vi "1_PatchCore_Eval.vi"(0 "Trained_Model_Paths":T6={"NNFE_Paths"={"CFG"=path "D:/bottle__25_02_07__21_20_24/bottle_NNFE__25_02_07__21_20_24.cfg", "BIN"=path "D:/bottle__25_02_07__21_20_24/bottle_NNFE__25_02_07__21_20_24.bin"}, "PatchCore_Paths"={"CFG"=path "D:/bottle__25_02_07__21_20_24/bottle_Patchcore__25_02_07__21_20_24.cfg", "BIN"=path "D:/bottle__25_02_07__21_20_24/bottle_MemBank__PS3_RP296_SR0.1_Size16.4k__25_02_07__21_20_24.bin"}}, 1 "NNFE_CFG":T10={"Input_Dims"={"C"=-1, "H"=-1, "W"=-1}, "mBatch"=1}, 3 "Feature_Scorer_Params":T8={"Nearest_Neihbours"=1, "Calculate Anomaly Map"=TRUE, "Gaussian_Blur"={"Kernel_Size"=33, "sigma"=4.0}}, 7 "Dataset_Path(Validation)":path=path "D:/MVTec/bottle/test", 9 "Ground_Truth_Folder_Path":path=path "D:/MVTec/bottle/ground_truth", 11 "error in":errorcluster, 12 "Device_Config.":T4={"Device"=enum."GPU", "GPU Id"=0}) -> (4 "Eval_Stats_File_Path":path=path "D:/bottle__25_02_07__21_20_24/PatchCore_Eval_Stats__25_02_07__21_20_46.cfg", 13 "Evaluation_Metrics(Pixel)":T1={"Scores(Good)"={"X Values"=[2.5187396848201753, 3.240138484239578, 3.9615372836589815, 4.682936083078385, 5.404334882497787, 6.125733681917191, 6.847132481336594, 7.568531280755996, 8.289930080175399, 9.011328879594803, 9.732727679014207, 10.454126478433608, 11.175525277853012, 11.896924077272416, 12.618322876691819, 13.339721676111221, 14.061120475530625, 14.782519274950028, 15.50391807436943, 16.225316873788834, 16.94671567320824, 17.668114472627643, 18.389513272047044, 19.110912071466444, 19.83231087088585, 20.553709670305253, 21.275108469724657, 21.99650726914406, 22.71790606856346, 23.439304867982866, 24.160703667402267, 24.88210246682167, 25.603501266241075, 26.32490006566048, 27.04629886507988, 27.767697664499284, 28.489096463918685, 29.21049526333809, 29.931894062757493, 30.653292862176897, 31.3746916615963, 32.096090461015706, 32.81748926043511, 33.538888059854514, 34.26028685927391, 34.981685658693316, 35.70308445811272, 36.42448325753212, 37.14588205695152, 37.867280856370925, 38.58867965579033, 39.310078455209734, 40.03147725462914, 40.75287605404854, 41.474274853467946, 42.19567365288734, 42.91707245230675, 43.63847125172615, 44.359870051145556, 45.08126885056496, 45.80266764998436, 46.52406644940376, 47.245465248823166, 47.96686404824257, 48.688262847661974, 49.40966164708138, 50.13106044650078, 50.85245924592019, 51.573858045339584, 52.29525684475899, 53.01665564417839, 53.7380544435978, 54.4594532430172, 55.1808520424366, 55.902250841856, 56.62364964127541, 57.34504844069481, 58.066447240114215, 58.78784603953362, 59.50924483895302, 60.23064363837243, 60.952042437791825, 61.67344123721123, 62.39484003663063, 63.11623883605004, 63.83763763546945, 64.55903643488884, 65.28043523430824, 66.00183403372765, 66.72323283314705, 67.44463163256646, 68.16603043198586, 68.88742923140526, 69.60882803082467, 70.33022683024407, 71.05162562966348, 71.77302442908287, 72.49442322850227, 73.21582202792167, 73.93722082734108], "Histogram: h(x)"=[90, 939, 2938, 5870, 8902, 11734, 15274, 18341, 21048, 26598, 31500, 33798, 32899, 32682, 35302, 38511, 44001, 47200, 57146, 83639, 108421, 109082, 88841, 61245, 37236, 23127, 12524, 6486, 3678, 1409, 910, 781, 568, 237, 213, 141, 123, 86, 0, 0, 0, 0, 0, 0, 0, 0, 0, 0, 0, 0, 0, 0, 0, 0, 0, 0, 0, 0, 0, 0, 0, 0, 0, 0, 0, 0, 0, 0, 0, 0, 0, 0, 0, 0, 0, 0, 0, 0, 0, 0, 0, 0, 0, 0, 0, 0, 0, 0, 0, 0, 0, 0, 0, 0, 0, 0, 0, 0, 0, 0]}, "Scores(Bad)"={"X Values"=[2.5187396848201753, 3.240138484239578, 3.9615372836589815, 4.682936083078385, 5.404334882497787, 6.125733681917191, 6.847132481336594, 7.568531280755996, 8.289930080175399, 9.011328879594803, 9.732727679014207, 10.454126478433608, 11.175525277853012, 11.896924077272416, 12.618322876691819, 13.339721676111221, 14.061120475530625, 14.782519274950028, 15.50391807436943, 16.225316873788834, 16.94671567320824, 17.668114472627643, 18.389513272047044, 19.110912071466444, 19.83231087088585, 20.553709670305253, 21.275108469724657, 21.99650726914406, 22.71790606856346, 23.439304867982866, 24.160703667402267, 24.88210246682167, 25.603501266241075, 26.32490006566048, 27.04629886507988, 27.767697664499284, 28.489096463918685, 29.21049526333809, 29.931894062757493, 30.653292862176897, 31.3746916615963, 32.096090461015706, 32.81748926043511, 33.538888059854514, 34.26028685927391, 34.981685658693316, 35.70308445811272, 36.42448325753212, 37.14588205695152, 37.867280856370925, 38.58867965579033, 39.310078455209734, 40.03147725462914, 40.75287605404854, 41.474274853467946, 42.19567365288734, 42.91707245230675, 43.63847125172615, 44.359870051145556, 45.08126885056496, 45.80266764998436, 46.52406644940376, 47.245465248823166, 47.96686404824257, 48.688262847661974, 49.40966164708138, 50.13106044650078, 50.85245924592019, 51.573858045339584, 52.29525684475899, 53.01665564417839, 53.7380544435978, 54.4594532430172, 55.1808520424366, 55.902250841856, 56.62364964127541, 57.34504844069481, 58.066447240114215, 58.78784603953362, 59.50924483895302, 60.23064363837243, 60.952042437791825, 61.67344123721123, 62.39484003663063, 63.11623883605004, 63.83763763546945, 64.55903643488884, 65.28043523430824, 66.00183403372765, 66.72323283314705, 67.44463163256646, 68.16603043198586, 68.88742923140526, 69.60882803082467, 70.33022683024407, 71.05162562966348, 71.77302442908287, 72.49442322850227, 73.21582202792167, 73.93722082734108], "Histogram: h(x)"=[0, 0, 0, 0, 0, 0, 0, 0, 0, 0, 0, 0, 0, 0, 0, 0, 0, 0, 0, 0, 0, 0, 0, 0, 3, 18, 4, 4, 22, 166, 350, 529, 712, 1080, 1390, 2090, 2510, 2735, 2990, 3683, 3643, 4025, 4368, 4354, 5075, 4848, 4451, 4310, 4479, 4659, 4932, 5114, 5826, 5988, 5477, 5336, 5670, 5902, 6292, 7002, 6961, 7000, 6738, 6629, 6889, 6684, 6682, 6438, 6484, 6148, 6044, 5899, 5338, 5008, 4726, 4469, 4002, 3233, 2677, 2298, 2183, 1919, 1568, 1056, 735, 519, 423, 414, 455, 561, 433, 377, 366, 353, 270, 185, 83, 74, 69, 64]}, "Eval Stats"={"Scores(Good)"={"Min"=2.1580403, "Max"=29.366932}, "Scores(Bad)"={"Min"=19.911945, "Max"=74.29792}, "# of Samples(Good)"=1003520, "# of Samples(Bad)"=242491, "AUROC"=0.9999726, "F1_Max"=0.994964, "Thrshld(F1_Max)"=25.554758, "Prec.(F1_Max)"=0.99552876, "Recall(F1_Max)"=0.9943998, "FPR(F1_Max)"=0.0010792012, "FNR(F1_Max)"=0.005600208}} {"Eval Stats"."Recall(F1_Max)" format="%#.5f"; "Eval Stats"."FPR(F1_Max)" format="%#.5f"; "Eval Stats"."FNR(F1_Max)" format="%#.5f"; "Eval Stats"."Prec.(F1_Max)" format="%#.5f"; "Eval Stats"."F1_Max" format="%#.5f"; "Eval Stats"."AUROC" format="%#.5f"; "Eval Stats"."Scores(Bad)"."Min" format="%#_5g"; "Eval Stats"."Scores(Good)"."Min" format="%#_5g"; "Eval Stats"."Thrshld(F1_Max)" format="%#_5f"}, 14 "Evaluation_Metrics(Image)":T1={"Scores(Good)"={"X Values"=[21.021667575836183, 21.57413511276245, 22.12660264968872, 22.679070186614993, 23.23153772354126, 23.78400526046753, 24.336472797393796, 24.88894033432007, 25.44140787124634, 25.993875408172606, 26.54634294509888, 27.098810482025144, 27.651278018951416, 28.203745555877685, 28.756213092803954, 29.308680629730226, 29.86114816665649, 30.413615703582764, 30.966083240509032, 31.5185507774353, 32.071018314361574, 32.62348585128784, 33.17595338821411, 33.728420925140384, 34.28088846206665, 34.83335599899292, 35.38582353591919, 35.93829107284546, 36.490758609771724, 37.043226146698, 37.59569368362427, 38.148161220550534, 38.70062875747681, 39.25309629440307, 39.805563831329344, 40.35803136825562, 40.91049890518188, 41.462966442108154, 42.01543397903442, 42.56790151596069, 43.120369052886964, 43.67283658981323, 44.2253041267395, 44.77777166366577, 45.33023920059204, 45.88270673751831, 46.43517427444458, 46.98764181137085, 47.540109348297115, 48.09257688522339, 48.64504442214966, 49.197511959075925, 49.7499794960022, 50.30244703292846, 50.854914569854735, 51.407382106781, 51.95984964370727, 52.512317180633545, 53.06478471755981, 53.61725225448608, 54.16971979141235, 54.72218732833862, 55.27465486526489, 55.82712240219116, 56.37958993911743, 56.932057476043695, 57.48452501296997, 58.03699254989624, 58.589460086822506, 59.14192762374878, 59.69439516067504, 60.246862697601316, 60.79933023452759, 61.35179777145385, 61.904265308380126, 62.45673284530639, 63.00920038223266, 63.561667919158936, 64.1141354560852, 64.66660299301148, 65.21907052993774, 65.77153806686401, 66.32400560379028, 66.87647314071654, 67.42894067764283, 67.98140821456909, 68.53387575149536, 69.08634328842163, 69.63881082534789, 70.19127836227418, 70.74374589920043, 71.2962134361267, 71.84868097305298, 72.40114850997924, 72.95361604690552, 73.50608358383178, 74.05855112075805, 74.61101865768433, 75.16348619461058, 75.71595373153687], "Histogram: h(x)"=[1, 0, 0, 8, 2, 2, 0, 1, 1, 0, 0, 2, 1, 0, 0, 1, 0, 0, 1, 0, 0, 0, 0, 0, 0, 0, 0, 0, 0, 0, 0, 0, 0, 0, 0, 0, 0, 0, 0, 0, 0, 0, 0, 0, 0, 0, 0, 0, 0, 0, 0, 0, 0, 0, 0, 0, 0, 0, 0, 0, 0, 0, 0, 0, 0, 0, 0, 0, 0, 0, 0, 0, 0, 0, 0, 0, 0, 0, 0, 0, 0, 0, 0, 0, 0, 0, 0, 0, 0, 0, 0, 0, 0, 0, 0, 0, 0, 0, 0, 0]}, "Scores(Bad)"={"X Values"=[21.021667575836183, 21.57413511276245, 22.12660264968872, 22.679070186614993, 23.23153772354126, 23.78400526046753, 24.336472797393796, 24.88894033432007, 25.44140787124634, 25.993875408172606, 26.54634294509888, 27.098810482025144, 27.651278018951416, 28.203745555877685, 28.756213092803954, 29.308680629730226, 29.86114816665649, 30.413615703582764, 30.966083240509032, 31.5185507774353, 32.071018314361574, 32.62348585128784, 33.17595338821411, 33.728420925140384, 34.28088846206665, 34.83335599899292, 35.38582353591919, 35.93829107284546, 36.490758609771724, 37.043226146698, 37.59569368362427, 38.148161220550534, 38.70062875747681, 39.25309629440307, 39.805563831329344, 40.35803136825562, 40.91049890518188, 41.462966442108154, 42.01543397903442, 42.56790151596069, 43.120369052886964, 43.67283658981323, 44.2253041267395, 44.77777166366577, 45.33023920059204, 45.88270673751831, 46.43517427444458, 46.98764181137085, 47.540109348297115, 48.09257688522339, 48.64504442214966, 49.197511959075925, 49.7499794960022, 50.30244703292846, 50.854914569854735, 51.407382106781, 51.95984964370727, 52.512317180633545, 53.06478471755981, 53.61725225448608, 54.16971979141235, 54.72218732833862, 55.27465486526489, 55.82712240219116, 56.37958993911743, 56.932057476043695, 57.48452501296997, 58.03699254989624, 58.589460086822506, 59.14192762374878, 59.69439516067504, 60.246862697601316, 60.79933023452759, 61.35179777145385, 61.904265308380126, 62.45673284530639, 63.00920038223266, 63.561667919158936, 64.1141354560852, 64.66660299301148, 65.21907052993774, 65.77153806686401, 66.32400560379028, 66.87647314071654, 67.42894067764283, 67.98140821456909, 68.53387575149536, 69.08634328842163, 69.63881082534789, 70.19127836227418, 70.74374589920043, 71.2962134361267, 71.84868097305298, 72.40114850997924, 72.95361604690552, 73.50608358383178, 74.05855112075805, 74.61101865768433, 75.16348619461058, 75.71595373153687], "Histogram: h(x)"=[0, 0, 0, 0, 0, 0, 0, 0, 0, 0, 0, 0, 0, 0, 0, 0, 0, 0, 0, 0, 0, 0, 0, 0, 0, 1, 0, 0, 0, 1, 1, 1, 1, 0, 0, 1, 0, 0, 0, 0, 1, 1, 0, 0, 1, 0, 0, 0, 1, 2, 1, 0, 1, 0, 2, 2, 0, 0, 0, 0, 1, 0, 2, 3, 0, 4, 0, 0, 1, 2, 2, 2, 3, 2, 3, 4, 1, 2, 2, 2, 2, 0, 0, 1, 0, 2, 0, 0, 0, 0, 0, 0, 1, 0, 1, 0, 1, 0, 0, 1]}, "Eval Stats"={"Scores(Good)"={"Min"=20.745434, "Max"=30.757803}, "Scores(Bad)"={"Min"=34.900276, "Max"=75.99219}, "# of Samples(Good)"=20, "# of Samples(Bad)"=63, "AUROC"=1.0, "F1_Max"=1.0, "Thrshld(F1_Max)"=30.810408, "Prec.(F1_Max)"=1.0, "Recall(F1_Max)"=1.0, "FPR(F1_Max)"=0.0, "FNR(F1_Max)"=0.0}} {"Eval Stats"."Recall(F1_Max)" format="%#.5f"; "Eval Stats"."FPR(F1_Max)" format="%#.5f"; "Eval Stats"."FNR(F1_Max)" format="%#.5f"; "Eval Stats"."Prec.(F1_Max)" format="%#.5f"; "Eval Stats"."F1_Max" format="%#.5f"; "Eval Stats"."AUROC" format="%#.5f"; "Eval Stats"."Scores(Bad)"."Min" format="%#_5g"; "Eval Stats"."Scores(Good)"."Min" format="%#_5g"; "Eval Stats"."Thrshld(F1_Max)" format="%#_5f"}, 15 "error out":errorcluster)   [LabVIEW 2020]
uses:
  PatchCore_AddOn/API/Controls/NNPC_Init_Custom_NN_CFG.ctl
  <vilib>/Ngene/Deep Learning Toolkit/Toolkit/NN_Data/API/NN_Dims(C,H,W).ctl
  PatchCore_AddOn/API/Controls/Feature_Scorer_Params.ctl
  PatchCore_AddOn/API/Controls/Gaussian_Blur.ctl
  PatchCore_AddOn/API/Controls/NNPC_Trained_Model_Paths.ctl
  PatchCore_AddOn/API/Controls/NN_Paths.ctl
  PatchCore_AddOn/API/Controls/NNPC_Device.ctl
  <vilib>/Ngene/Deep Learning Toolkit/Toolkit/NN_Network/Controls/NN_Device.ctl
  PatchCore_AddOn/API/Controls/Evaluation_Metrics.ctl
  PatchCore_AddOn/API/Controls/Eval_Results.ctl
  PatchCore_AddOn/API/Controls/MinMax.ctl
  subVIs/Dataset_Reader/Controls/Read_Options.ctl
  PatchCore_AddOn/API/Controls/Eval_Config.ctl
  subVIs/Dataset_Reader/Controls/ImRead_PreProcessing_Options.ctl
  PatchCore_AddOn/Low_Level/Controls/Normalization_Type.ctl
  PatchCore_AddOn/API/NNPC_Predict/NNPC_Predict(Dataset).vi
  <vilib>/Ngene/Deep Learning Toolkit/Toolkit/NN_Data/subVIs/Dataset_Destroy/NN_Dataset_Destroy(In3D_Out3D).vi
  PatchCore_AddOn/PatchCore_AddOn.lvlib
  <vilib>/Ngene/Deep Learning Toolkit/Toolkit/Deep_Learning_Toolkit_by_Ngene.lvlib
panel:
  out "dT_Init_Infer.":dbl=2.254286299998057 format="%#_4p"
  out "dT_Predict":dbl=0.6033489999972517 format="%#_4p"
  out "dT_Total":dbl=5.14764589999686 format="%#_4p"
  in  "Dest. Path":path
  out "dT_Eval":dbl=0.392645400002948 format="%#_4p"
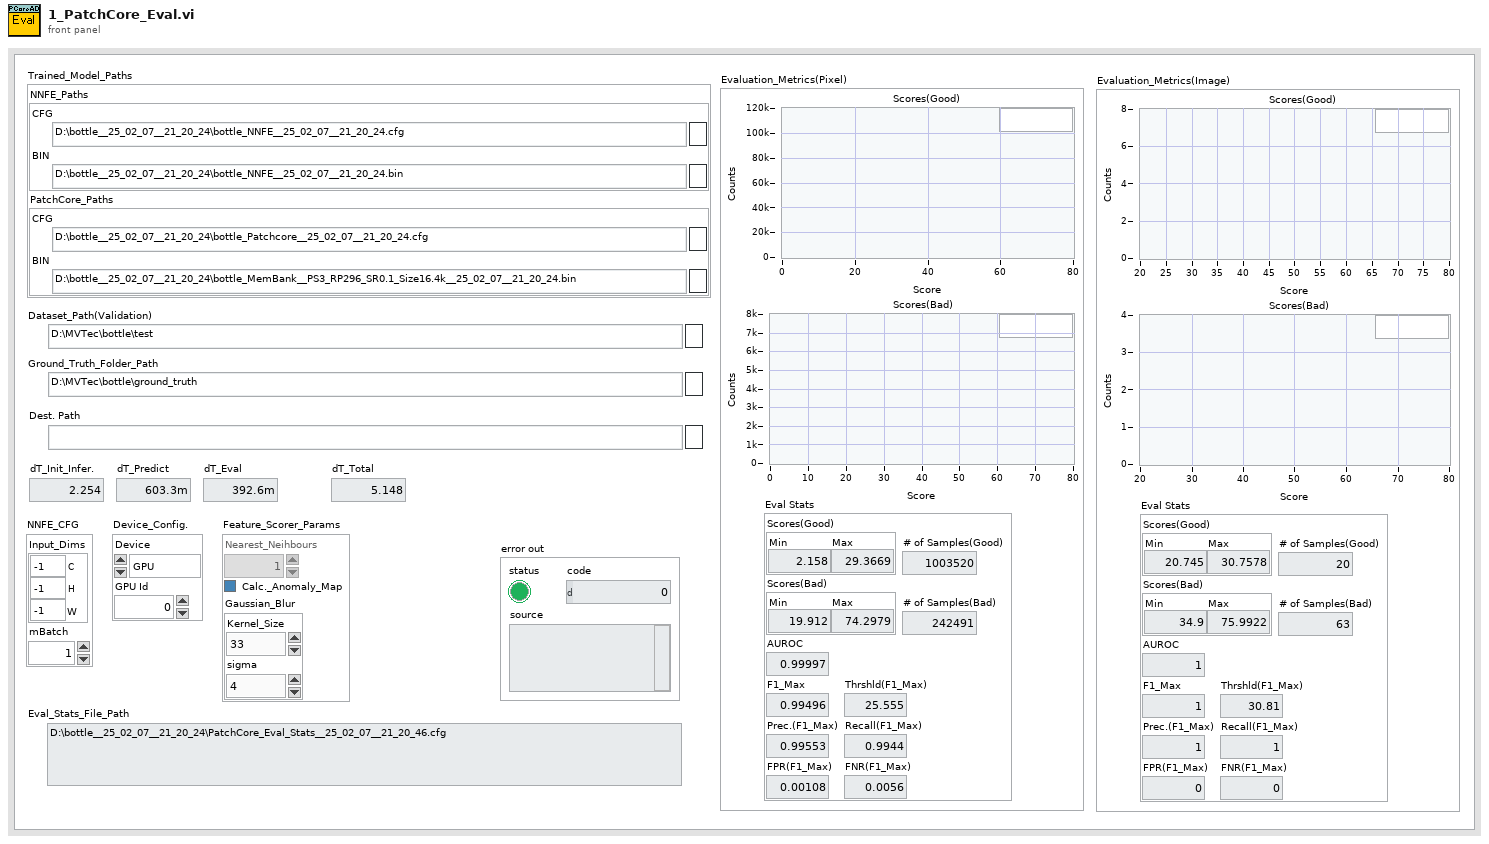
[diagram p1: front panel]
types:
  T1 = typedef "PatchCore_AddOn.lvlib/Evaluation_Metrics.ctl" = cluster{"Scores(Good)":cluster{"X Values":dbl[], "Histogram: h(x)":i32[]}, "Scores(Bad)":cluster{"X Values":dbl[], "Histogram: h(x)":i32[]}, "Eval Stats":T2}
  T2 = typedef "PatchCore_AddOn.lvlib/Eval_Results.ctl" = cluster{"Scores(Good)":T3, "Scores(Bad)":T3, "# of Samples(Good)":i32, "# of Samples(Bad)":i32, "AUROC":sgl, "F1_Max":sgl, "Thrshld(F1_Max)":sgl, "Prec.(F1_Max)":sgl, "Recall(F1_Max)":sgl, "FPR(F1_Max)":sgl, "FNR(F1_Max)":sgl}
  T3 = typedef "PatchCore_AddOn.lvlib/MinMax.ctl" = cluster{"Min":sgl, "Max":sgl}
  T4 = typedef "PatchCore_AddOn.lvlib/NNPC_Device.ctl" = cluster{"Device":T5, "GPU Id":i32}
  T5 = typedef "Deep_Learning_Toolkit_by_Ngene.lvlib/NN_Device.ctl" = enum16{"CPU", "GPU"}
  T6 = typedef "PatchCore_AddOn.lvlib/NNPC_Trained_Model_Paths.ctl" = cluster{"NNFE_Paths":T7, "PatchCore_Paths":T7}
  T7 = typedef "PatchCore_AddOn.lvlib/NN_Paths.ctl" = cluster{"CFG":path, "BIN":path}
  T8 = typedef "PatchCore_AddOn.lvlib/Feature_Scorer_Params.ctl" = cluster{"Nearest_Neihbours":i32, "Calculate Anomaly Map":bool, "Gaussian_Blur":T9}
  T9 = typedef "PatchCore_AddOn.lvlib/Gaussian_Blur.ctl" = cluster{"Kernel_Size":i32, "sigma":sgl}
  T10 = typedef "PatchCore_AddOn.lvlib/NNPC_Init_Custom_NN_CFG.ctl" = cluster{"Input_Dims":T11, "mBatch":i32}
  T11 = typedef "Deep_Learning_Toolkit_by_Ngene.lvlib/NN_Dims(C,H,W).ctl" = cluster{"C":i32, "H":i32, "W":i32}
  T12 = typedef "PatchCore_AddOn.lvlib/Eval_Config.ctl" = cluster{"Extract Good Pixels from Bad":bool, "# bins":i32}
  T13 = typedef "Read_Options.ctl" = cluster{"Read Bads?":bool, "Read GTs?":bool, "Calc. DS Stats?":bool}
  T14 = typedef "ImRead_PreProcessing_Options.ctl" = cluster{"Image Type":T15, "Normalization Type":T16, "Interpolation Type":u32}
  T15 = typedef "Image Type" = u32
  T16 = typedef "PatchCore_AddOn.lvlib/Normalization_Type.ctl" = enum16{"Standardize(DS_Stats)", "Standardize(Image_Stats)"}
  T17 = typedef "PatchCore_AddOn.lvlib/NNPC_Instance.ctl" = cluster{"Dataset_Stats":T18, "NN":T20, "Device_Config.":T4, "PatchCore_Init_CFG":T35, "Coreset Params":T37, "MemBank_Data":T39}
  T18 = typedef "PatchCore_AddOn.lvlib/NNPC_DS_Stats.ctl" = cluster{"means":T19, "vars":T19, "DS_Size":i32}
  T19 = typedef "PatchCore_AddOn.lvlib/Image_Stats_RGB.ctl" = cluster{"R":sgl, "G":sgl, "B":sgl}
  T20 = typedef "Deep_Learning_Toolkit_by_Ngene.lvlib/NN.ctl" = cluster{"Name":string, "No of Layers":i32, "mBatch":i32, "Layers":T21[], "Dimty":T22, "Dims_In":T11, "Dims_Out":T11, "Working_Dir":path, "Train?":bool, "Train_Params":T23, "LR_Update_Policy":T26, "Session Data":T28, "Ground_truth":T29, "NNg_hdls":T30, "NN_Device":T5, "GPU Id":i32, "Labels":string[], "Receptive Field":T31[], "Loss_Type":T32, "Loss_Cfg_Prms":variant, "NNG_WS":T33}
  T21 = typedef "Deep_Learning_Toolkit_by_Ngene.lvlib/NN_Layer_ref.ctl" = refnum<data-value>
  T22 = typedef "Deep_Learning_Toolkit_by_Ngene.lvlib/NN_In_Out_Dim-ty.ctl" = enum8{"In1D_Out1D", "In3D_Out1D", "In3D_Out3D", "In3D_OutBBox"}
  T23 = typedef "Deep_Learning_Toolkit_by_Ngene.lvlib/NN_Train_Params.ctl" = cluster{"Optimizer":T24, "Beta_1":sgl, "Beta_2":sgl, "Weight Decay(L1)":sgl, "Weight Decay(L2)":sgl, "Data_Sampling":T25}
  T24 = typedef "Deep_Learning_Toolkit_by_Ngene.lvlib/NN_Train_Optimizer.ctl" = enum16{"SGD", "Adam", "Adagrad", "Adadelta", "RMSProp", "Nesterov"}
  T25 = typedef "Deep_Learning_Toolkit_by_Ngene.lvlib/NN_Train_Data_Sampling.ctl" = enum16{"Random", "Sequential"}
  T26 = typedef "Deep_Learning_Toolkit_by_Ngene.lvlib/NN_LR_Policy_Cfg.ctl" = cluster{"Policy_Type":T27, "LR0":dbl, "k":sgl, "WarmUp_Policy":enum16{"Step", "Ramp"}, "WarmUp_Iter":i32, "WarmUp_Ratio":sgl}
  T27 = typedef "Deep_Learning_Toolkit_by_Ngene.lvlib/NN_LR_Policy_Type.ctl" = enum16{"Manual", "Step", "Exp", "1/t"}
  T28 = typedef "Deep_Learning_Toolkit_by_Ngene.lvlib/NN_Train_Session_Data.ctl" = cluster{"Epochs":sgl, "Tot_Iter":i32, "LR":sgl, "LR_iter":i32}
  T29 = typedef "Deep_Learning_Toolkit_by_Ngene.lvlib/NN_Ground_truth.ctl" = cluster{"Y":variant}
  T30 = typedef "Deep_Learning_Toolkit_by_Ngene.lvlib/nng_cuda_handles.ctl" = cluster{"cudnn":u64, "cublas":u64, "stream":u64, "curand":u64}
  T31 = typedef "Deep_Learning_Toolkit_by_Ngene.lvlib/NN_Dims(V,H).ctl" = cluster{"V":i32, "H":i32}
  T32 = typedef "Deep_Learning_Toolkit_by_Ngene.lvlib/NN_Loss_Type.ctl" = enum16{"None", "MSE", "CrossEntropy", "YOLO_v2", "YOLO_v4"}
  T33 = typedef "Deep_Learning_Toolkit_by_Ngene.lvlib/NNG_WS.ctl" = cluster{"NNG_WS_Mem":T34, "Max_WS_Size":i64}
  T34 = typedef "Deep_Learning_Toolkit_by_Ngene.lvlib/NNg_WS_Mem_DVR.ctl" = refnum<data-value>
  T35 = typedef "PatchCore_AddOn.lvlib/NNPC_Init_CFG.ctl" = cluster{"BackBone":T36, "Out_Layers_Names":string[], "Patch_Size":u32}
  T36 = typedef "PatchCore_AddOn.lvlib/NNPC_BackBone_Selector.ctl" = enum16{"WRN_50_2_L2L3"}
  T37 = typedef "PatchCore_AddOn.lvlib/NNPC_Coreset_Params.ctl" = cluster{"Name":string, "Sampling_Ratio":sgl, "Startd_idx":i32, "Random_Proj?":bool, "Rnd. Proj. Params":T38}
  T38 = typedef "PatchCore_AddOn.lvlib/NNPC_Random_Projection_CFG.ctl" = cluster{"Proj._Dim.":i32, "Epsilon":sgl, "Seed":i32}
  T39 = typedef "PatchCore_AddOn.lvlib/MemBank_and_Norm_Variants.ctl" = cluster{"MemBank":variant, "MemBank Norm":variant}
  T40 = typedef "Deep_Learning_Toolkit_by_Ngene.lvlib/NN_DataSet(In3D_Out3D).ctl" = cluster{"Dataset_Size":i32, "Dims_In":T11, "Labels":string[], "File Paths":path[], "Outputs Ref.":T41, "Inputs Ref.":variant, "Dims_Out":T11}
  T41 = typedef "Deep_Learning_Toolkit_by_Ngene.lvlib/NN_Data_ref(4D_SGL).ctl" = refnum<data-value>
  T42 = typedef "imagedata.ctl" = cluster{"image type":i32, "image depth":i32, "image":u8[], "mask":u8[], "colors":u32[], "Rectangle":cluster{"left":i16, "top":i16, "right":i16, "bottom":i16}}
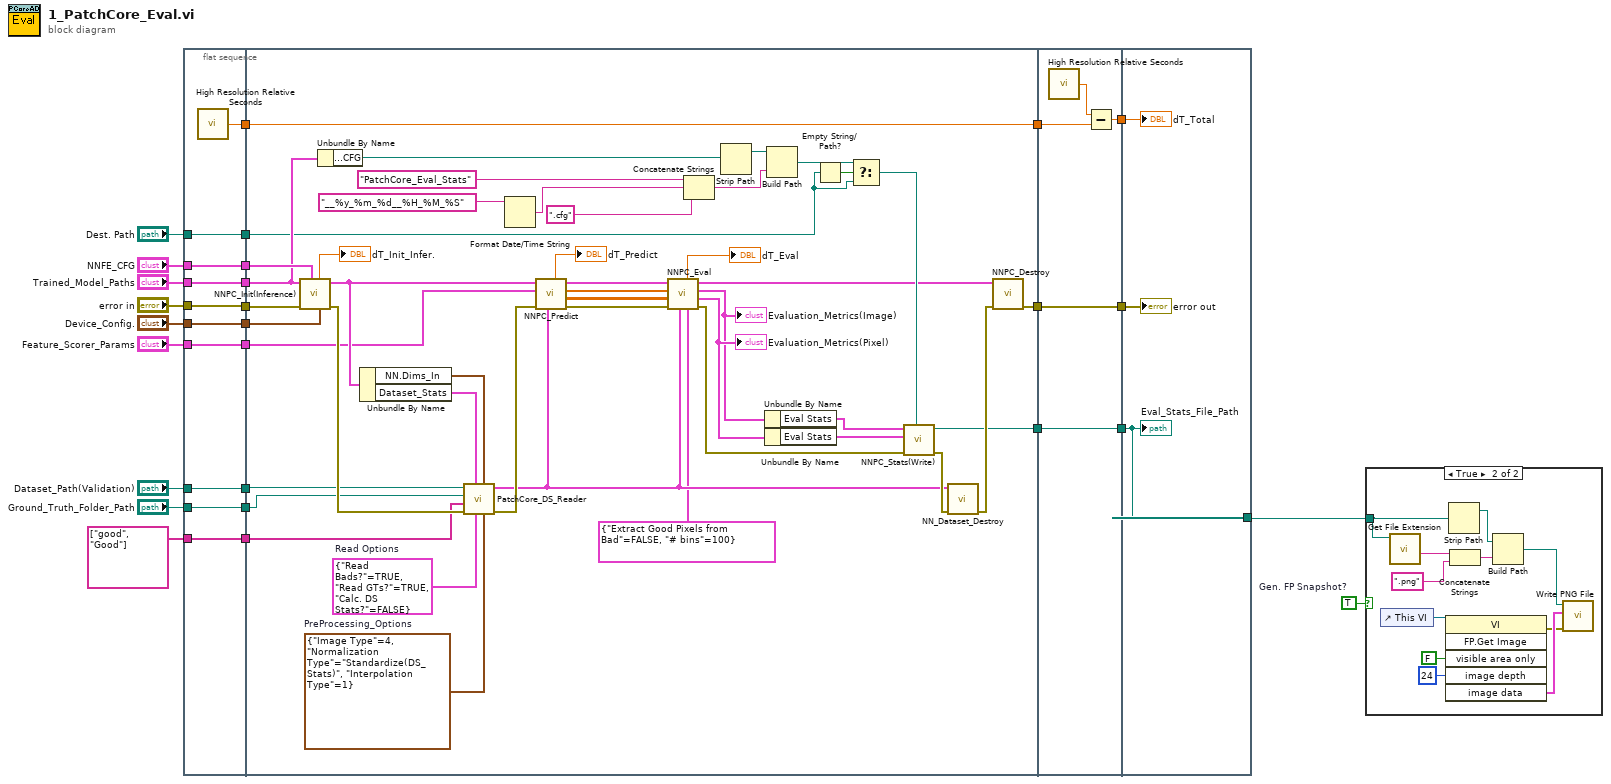
[diagram p0: block diagram]
diagram:
  w8 = TRUE  # Gen. FP Snapshot?
  n1 = flat-sequence {
    tunnel: "Dest. Path" -> [w31]
    tunnel: "Ground_Truth_Folder_Path" -> [w32]
    tunnel: "Feature_Scorer_Params" -> [w33]
    tunnel: "NNFE_CFG" -> [w34]
    tunnel: string[] ["good", "Good"] ("Good Folder Name") -> [w35]
    tunnel: "Dataset_Path(Validation)" -> [w36]
    tunnel: "Trained_Model_Paths" -> [w37]
    tunnel: [w37] -> w20
    tunnel: [w36] -> w19
    tunnel: [w35] -> w18
    tunnel: [w34] -> w17
    tunnel: [w33] -> w16
    tunnel: [w32] -> w15
    tunnel: [w31] -> w14
    tunnel: [w30] -> w12
    tunnel: [w29] -> w10
    tunnel: "Device_Config." -> [w29]
    tunnel: [w28] -> w2
    tunnel: "error in" -> [w28]
    tunnel: [w80] -> w21
    tunnel: w20 -> [w65]
    tunnel: w19 -> [w55]
    tunnel: w18 -> [w53]
    tunnel: w17 -> [w79]
    tunnel: w16 -> [w50]
    tunnel: w15 -> [w54]
    tunnel: w14 -> [w56]
    tunnel: [w69] -> w13
    tunnel: w12 -> [w69]
    tunnel: w10 -> [w64]
    tunnel: [w63] -> w7
    tunnel: w2 -> [w62]
    tunnel: w21 -> [w88]
    tunnel: w13 -> [w86]
    tunnel: w7 -> [w84]
    tunnel: [w88] -> w5
    tunnel: [w85] -> w4
    tunnel: [w84] -> w3
    tunnel: [w91] -> w6
    tunnel: w5 -> [w90]
    tunnel: w4 -> [w89]
    tunnel: w3 -> [w91]
    frame #0 {
      n2 = call <vilib>:"High Resolution Relative Seconds.vi"() -> ("relative seconds"=w30:dbl)
    }
    frame #1 {
      w39 = T13 {"Read Bads?"=TRUE, "Read GTs?"=TRUE, "Calc. DS Stats?"=FALSE}  # Read Options
      w43 = T14 {"Image Type"=4, "Normalization Type"=enum."Standardize(DS_Stats)", "Interpolation Type"=1}  # PreProcessing_Options
      n3 = call "NNPC_Init(Inference).vi"("Device_Config."=w64, "NNFE_Custom_CFG"=w79, "error in"=w62, "NNFE PatchCore Paths"=w65) -> ("error out"=w81:errorcluster, "PCore_Instance out"=w78:T17, "dT_Init_Inference"=→"dT_Init_Infer.":dbl)  [unwired: 5 in]
      n4 = Unbundle By Name(w65) -> ("NNFE_Paths.CFG"=w75:path)
      n5 = Unbundle By Name(w78) -> ("NN.Dims_In"=w51:T11, "Dataset_Stats"=w52:T18)
      n6 = call "PatchCore_DS_Reader.vi"("PreProcessing_Options"=w43, "Input3D_Custom_Dims"=w51, "Read Options"=w39, "Dataset_Stats In"=w52, "error in (no error)"=w81, "Good Unique Labels"=w53, "GT Folder Path"=w54, "Image File Paths"=w55) -> ("error out"=w49:errorcluster, "Dataset(In3D_Out3D)"=w42:T40)  [unwired: 2 out]
      n7 = Format Date/Time String(time format string (%c)="__%y_%m_%d__%H_%M_%S") -> (date/time string=w67:string)  [unwired: 2 in]
      n8 = call-poly "NNPC_Predict.vi"("Dataset"=w42, "error in (no error)"=w49, "Feature Scorer Params"=w50, "PCore_Instance in"=w78) -> ("error out"=w45:errorcluster, "anomaly maps"=w44:sgl[][][], "pred scores"=w46:sgl[], "PCore_Instance out"=w48:T17, "dT_Predict"=→"dT_Predict":dbl)  [unwired: 3 in]
      n9 = call "NNPC_Eval.vi"("Eval Config"=T12 {"Extract Good Pixels from Bad"=FALSE, "# bins"=100}, "Dataset(In3D_Out3D)"=w42, "error in"=w45, "anomaly maps"=w44, "pred scores"=w46, "PCore_Instance in"=w48) -> ("error out"=w77:errorcluster, "Evaluation_Metrics(Pixel)"=w60:T1, "Evaluation_Metrics(Image)"=w58:T1, "PCore_Instance out"=w47:T17, "dT_Eval"=→"dT_Eval":dbl)  [unwired: 1 in]
      "Evaluation_Metrics(Image)" <- w58
      "Evaluation_Metrics(Pixel)" <- w60
      n10 = Concatenate Strings("PatchCore_Eval_Stats" ("string"), w67, ".cfg" ("string")) -> (w74:string)
      n11 = Strip Path(path=w75) -> (stripped path=w66:path)  [unwired: 1 out]
      n12 = Unbundle By Name(w58) -> ("Eval Stats"=w57:T2)
      n13 = Unbundle By Name(w60) -> ("Eval Stats"=w59:T2)
      n14 = Build Path(base path=w66, name or relative path=w74) -> (appended path=w72:path)
      n15 = Empty String/Path?(string/path=w56) -> (empty?=w76:bool)
      n16 = Select(t=w72, s=w76, f=w56) -> (s? t:f=w70:path)
      n17 = call "NNPC_Stats(Write).vi"("CFG File Path"=w70, "error in (no error)"=w77, "Pixel Results"=w59, "Image Results"=w57) -> ("error out"=w82:errorcluster, "CFG File Path"=w63:path)  [unwired: 6 in]
      n18 = call-poly <vilib>:"NN_Dataset_Destroy.vi"("error in (no error)"=w82, "Dataset(In3D_Out3D)"=w42) -> ("error out"=w83:errorcluster)  [unwired: 9 in]
      n19 = call "NNPC_Destroy.vi"("error in"=w83, "PCore_Instance in"=w47) -> ("error out"=w80:errorcluster)  [unwired: 9 in]
    }
    frame #2 {
      n20 = call <vilib>:"High Resolution Relative Seconds.vi"() -> ("relative seconds"=w87:dbl)
      n21 = Subtract(x=w87, y=w86) -> (x-y=w85:dbl)
    }
    frame #3 {
      "dT_Total" <- w89
      "error out" <- w90
      "Eval_Stats_File_Path" <- w91
    }
  }
  n22 = case shown="True" w8 {
    tunnel: w6 -> [_ w92]
    frame False {
    }
    frame True {
      n23 = control-ref of="This VI"() -> (w102:refnum<vi>)
      n24 = call <vilib>:"Get File Extension.vi"("file"=w92) -> ("filename without extension"=w97:string)  [unwired: 6 in, 4 out]
      n25 = invoke class="VI" method="FP.Get Image"(reference=w102, "visible area only"=FALSE ("Visible Area Only"), "image depth"=24 ("Image Depth")) -> (error out=w98:errorcluster, "image data"=w99:T42)  [unwired: 3 in, 4 out]
      n26 = Strip Path(path=w92) -> (stripped path=w94:path)  [unwired: 1 out]
      n27 = Concatenate Strings(w97, ".png" ("string")) -> (w95:string)
      n28 = Build Path(base path=w94, name or relative path=w95) -> (appended path=w93:path)
      n29 = call <vilib>:"Write PNG File.vi"("error in (no error)"=w98, "image data"=w99, "path to PNG file"=w93) -> ()  [unwired: 7 in, 2 out]
    }
  }
